vi "TCV_Query.vi"(0 "System no.":i32=1 min=1 max=4 step=1, 2 "Axes to query":string[](array[string]), 3 "All axes?":bool, 4 "Axis identifier?":bool=TRUE, 5 "error in":errorcluster) -> (14 "Velocity":dbl[](array[numeric]) format="%.6f", 19 "error out":errorcluster)   [LabVIEW 2020]
doc: "Returns current commanded velocity for specified axes. In contrast to VEL?, during acceleration and deceleration TCV? reports the value currently produced by the trajectory generator. The sign of the returned value depends on the commanded direction of motion. If the velocity of the axis is controlled by an axis of a Human Interface Device (i.e. HI control is activated, see HIA and HIN), TCV? returns the current value according to the deflection of the HID axis, and VEL? returns the maximum velocity set by the corresponding parameter or VEL.\n\nC-867, Mercury_GCS: If All axes? = TRUE, then Axis identifier? can be FALSE. Velocity unit is mm/s. \n\nC-877, C-884, C-891: If All axes? = TRUE, then Axis identifier? can be FALSE. Velocity unit is mm/s."
panel:
  # "Returns current commanded velocity for specified axes."
  # "If all axes: use"
  # "Query"
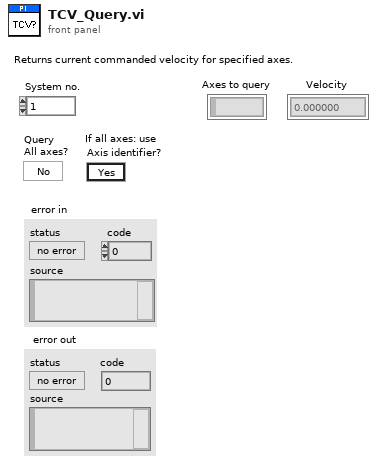
[diagram p1: front panel]
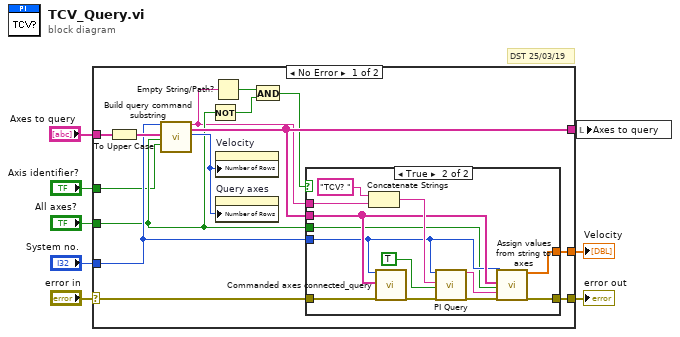
[diagram p0: block diagram]
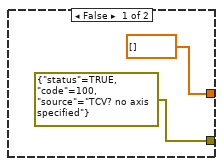
[diagram p2: hidden frame]
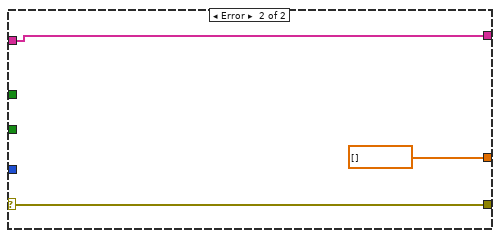
[diagram p3: hidden frame]
diagram:
  # "DST 25/03/19"
  n1 = case shown="No Error" "error in" {
    selector: "error in" -> [w9 w39]
    tunnel: [w22 dbl[] [] ("Values")] -> w8
    tunnel: "Axes to query" -> [w21 w38]
    tunnel: [w20 w39] -> w6
    tunnel: "Axis identifier?" -> [w13 _]
    tunnel: "System no." -> [w15 _]
    tunnel: [w17 w38] -> w3
    tunnel: "All axes?" -> [w14 _]
    frame No Error {
      n2 = To Upper Case(1:w21) -> (0:w19:string[])
      n3 = call "Build query command substring.vi"("System no."=w15, "Axes to query in"=w19, "Query\nAll axes?"=w14, "For all axes: use\nAxis identifier?"=w13) -> ("Command substring"=w11:string, "Axes to query out"=w17:string[], "Number of rows"=w18:u32)  [unwired: 2 in, 11 out]
      n4 = Not(x=w14) -> (.not. x?=w16:bool)
      n5 = Empty String/Path?(string/path=w11) -> (empty?=w10:bool)
      n6 = property on="Velocity" class="Arr (strict)"("Number of Rows"=w18) -> ()  [unwired: 2 in, 2 out]
      n7 = property on="Query axes" class="Arr (strict)"("Number of Rows"=w18) -> ()  [unwired: 2 in, 2 out]
      n8 = And(x=w10, y=w16) -> (x .and. y?=w12:bool)
      n9 = case shown="True" w12 {
        tunnel: [dbl[] [] ("Values") w34] -> w22
        tunnel: w9 -> [_ w33]
        tunnel: [errorcluster {"status"=TRUE, "code"=100, "source"="TCV? no axis specified"} ("error out") w25] -> w20
        tunnel: w11 -> [_ w32]
        tunnel: w17 -> [_ w31]
        tunnel: w15 -> [_ w29]
        tunnel: w14 -> [_ w28]
        frame False {
        }
        frame True {
          n10 = Concatenate Strings("TCV? ", w32) -> (w35:string)
          n11 = call "Commanded axes connected_query.vi"("System no."=w29, "Commanded axes"=w31, "error in"=w33) -> ("error out"=w30:errorcluster)  [unwired: 1 in, 15 out]
          n12 = call "PI Query.vi"("System no."=w29, "String to send"=w35, "Attach termination char.?"=TRUE ("Attach Linefeed?"), "error in"=w30) -> ("String read"=w27:string, "error out"=w26:errorcluster)  [unwired: 3 in, 11 out]
          n13 = call "Assign values from string to axes.vi"("System no."=w29, "Queried axes"=w31, "All axes queried?"=w28, "Input String"=w27, "error in"=w26) -> ("Values"=w34:dbl[], "error out"=w25:errorcluster)  [unwired: 4 in, 9 out]
        }
      }
    }
    frame Error {
    }
  }
  "error out" <- w6
  "Velocity" <- w8
  n14 = local write "Axes to query"(w3) -> ()
